vi "Get Font Height.vi"(8 "error in (no error)":errorcluster caption="错误输入（无错误）", 11 "Font 输入":refnum<class "Font.lvclass"> caption="DNL_LabVIEW Object in") -> (0 "error out":errorcluster caption="错误输出", 2 "GetHeight":sgl, 3 "Font 输出":refnum<class "Font.lvclass"> caption="DNL_LabVIEW Object out")   [LabVIEW 2011, in "Font.lvclass"]
uses:
  Font.lvclass
  Font.lvclass/Font.ctl
  System.Drawing
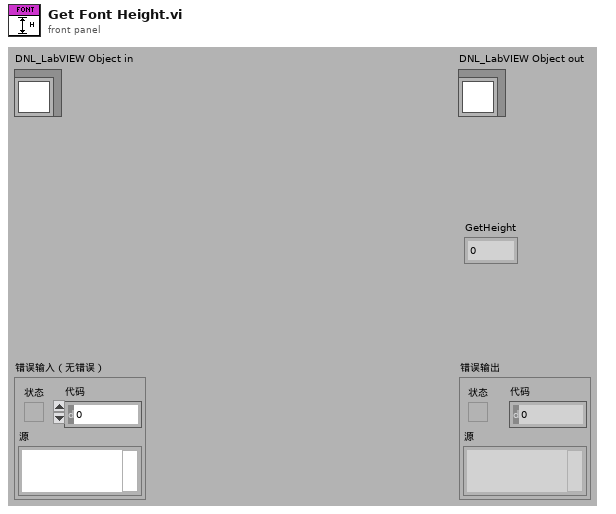
[diagram p1: front panel]
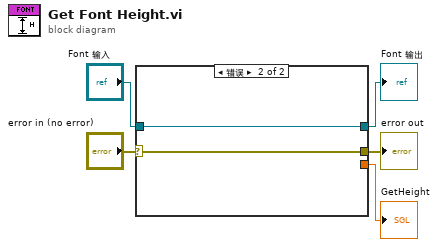
[diagram p0: block diagram]
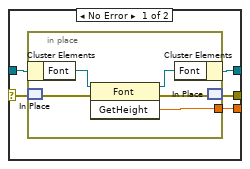
[diagram p2: hidden frame]
diagram:
  n1 = case shown="错误" "error in (no error)" {
    selector: "error in (no error)" -> [w9 w17]
    tunnel: [w8 w17] -> w4
    tunnel: [w7 w16] -> w2
    tunnel: "Font 输入" -> [w10 w16]
    tunnel: [w6 _] -> w1
    frame No Error {
      n2 = in-place {
        in-place-border: [w13] -> w6
        n3 = in-place-cluster #1(w10) -> ("Font"=w15:refnum<k24>)
        n4 = in-place-match #2(w9) -> (w12:errorcluster)
        n5 = invoke class="Font" method="GetHeight"(reference=w15, error in=w12) -> (reference out=w14:refnum<k24>, error out=w11:errorcluster, "GetHeight"=w13:sgl)  [unwired: 1 in]
        n6 = in-place-cluster #1("Font"=w14) -> (w7:refnum<class "Font.lvclass">)
        n7 = in-place-match #2(w11) -> (w8:errorcluster)
      }
    }
    frame Error {
    }
  }
  "error out" <- w4
  "Font 输出" <- w2
  "GetHeight" <- w1
